vi "Connector 1 DI Engine Sim 2.vi"() -> (3 "Packet":u64)   [LabVIEW 2014]
uses:
  <vilib>/rvi/eio/common/nirviEmuTemplateMethod_errors.vi
  <vilib>/eio/EIONode/EIONode.xnode
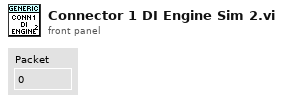
[diagram p1: front panel]
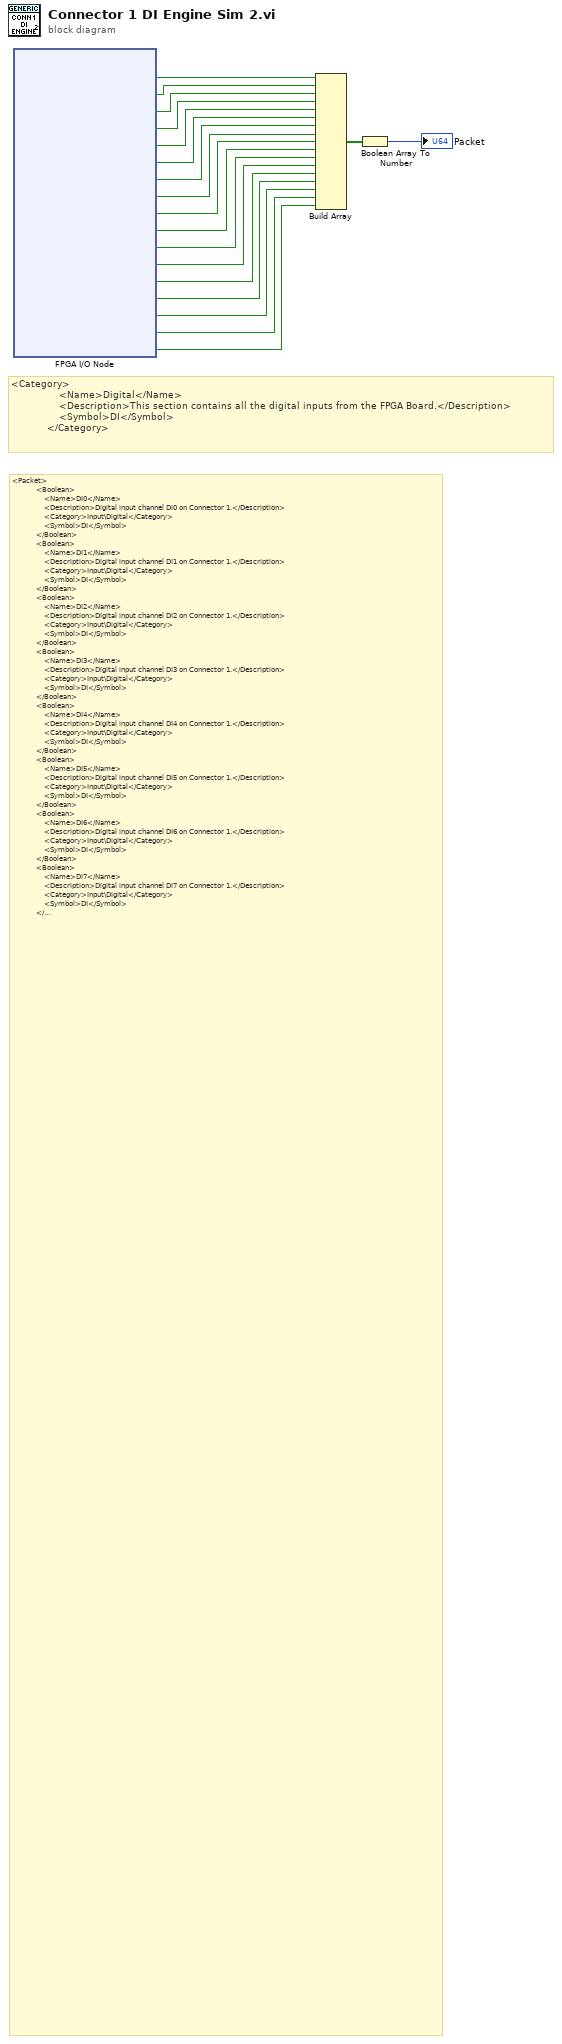
[diagram p0: block diagram]
diagram:
  # "<Packet>\n            <Boolean>\n                <Name>DI0</Name>\n                <Description>Digital input channel DI0 on Connector 1.</Description>\n                <Category>Input\\Digital</Category>\n                <Symbol>DI</Symbol>\n            </Boolean>\n            <Boolean>\n                <Name>DI1</Name>\n                <Description>Digital input channel DI1 on Connector 1.</Description>\n                <Category>Input\\Digital</Category>\n                <Symbol>DI</Symbol>\n            </Boolean>\n            <Boolean>\n                <Name>DI2</Name>\n                <Description>Digital input channel DI2 on Connector 1.</Description>\n                <Category>Input\\Digital</Category>\n                <Symbol>DI</Symbol>\n            </Boolean>\n            <Boolean>\n                <Name>DI3</Name>\n                <Description>Digital input channel DI3 on Connector 1.</Description>\n                <Category>Input\\Digital</Category>\n                <Symbol>DI</Symbol>\n            </Boolean>\n            <Boolean>\n                <Name>DI4</Name>\n                <Description>Digital input channel DI4 on Connector 1.</Description>\n                <Category>Input\\Digital</Category>\n                <Symbol>DI</Symbol>\n            </Boolean>\n            <Boolean>\n                <Name>DI5</Name>\n                <Description>Digital input channel DI5 on Connector 1.</Description>\n                <Category>Input\\Digital</Category>\n                <Symbol>DI</Symbol>\n            </Boolean>\n            <Boolean>\n                <Name>DI6</Name>\n                <Description>Digital input channel DI6 on Connector 1.</Description>\n                <Category>Input\\Digital</Category>\n                <Symbol>DI</Symbol>\n            </Boolean>\n            <Boolean>\n                <Name>DI7</Name>\n                <Description>Digital input channel DI7 on Connector 1.</Description>\n                <Category>Input\\Digital</Category>\n                <Symbol>DI</Symbol>\n            </Boolean>\n            <Boolean>\n                <Name>DI8</Name>\n                <Description>Digital input channel DI8 on Connector 1.</Description>\n                <Category>Input\\Digital</Category>\n                <Symbol>DI</Symbol>\n            </Boolean>\n            <Boolean>\n                <Name>DI9</Name>\n                <Description>Digital input channel DI9 on Connector 1.</Description>\n                <Category>Input\\Digital</Category>\n                <Symbol>DI</Symbol>\n            </Boolean>\n            <Boolean>\n                <Name>DI10</Name>\n                <Description>Digital input channel DI10 on Connector 1.</Description>\n                <Category>Input\\Digital</Category>\n                <Symbol>DI</Symbol>\n            </Boolean>\n            <Boolean>\n                <Name>DI11</Name>\n                <Description>Digital input channel DI11 on Connector 1.</Description>\n                <Category>Input\\Digital</Category>\n                <Symbol>DI</Symbol>\n            </Boolean>\n            <Boolean>\n                <Name>DI12</Name>\n                <Description>Digital input channel DI12 on Connector 1.</Description>\n                <Category>Input\\Digital</Category>\n                <Symbol>DI</Symbol>\n            </Boolean>\n            <Boolean>\n                <Name>DI13</Name>\n                <Description>Digital input channel DI13 on Connector 1.</Description>\n                <Category>Input\\Digital</Category>\n                <Symbol>DI</Symbol>\n            </Boolean>\n            <Boolean>\n                <Name>DI14</Name>\n                <Description>Digital input channel DI14 on Connector 1.</Description>\n                <Category>Input\\Digital</Category>\n                <Symbol>DI</Symbol>\n            </Boolean>\n            <Boolean>\n                <Name>DI15</Name>\n                <Description>Digital input channel DI15 on Connector 1.</Description>\n                <Category>Input\\Digital</Category>\n                <Symbol>DI</Symbol>\n            </Boolean>\n            <Boolean>\n                <Name>DI37</Name>\n                <Description>Digital input channel DI37 on Connector 1.</Description>\n                <Category>Input\\Digital</Category>\n                <Symbol>DI</Symbol>\n            </Boolean>\n        </Packet>"
  # "<Category>\n                <Name>Digital</Name>\n                <Description>This section contains all the digital inputs from the FPGA Board.</Description>\n                <Symbol>DI</Symbol>\n            </Category>"
  n1 = xnode "FPGA I/O Node"() -> ("Connector1/DIO0"=w19:bool, "Connector1/DIO1"=w18:bool, "Connector1/DIO2"=w17:bool, "Connector1/DIO3"=w16:bool, "Connector1/DIO4"=w15:bool, "Connector1/DIO5"=w14:bool, "Connector1/DIO6"=w13:bool, "Connector1/DIO7"=w12:bool, "Connector1/DIO8"=w11:bool, "Connector1/DIO9"=w10:bool, "Connector1/DIO10"=w9:bool, "Connector1/DIO11"=w8:bool, "Connector1/DIO12"=w7:bool, "Connector1/DIO13"=w6:bool, "Connector1/DIO14"=w5:bool, "Connector1/DIO15"=w4:bool, "Connector1/DIO37"=w3:bool)  [unwired: 17 in, 17 out]
  n2 = Build Array(w19, w18, w17, w16, w15, w14, w13, w12, w11, w10, w9, w8, w7, w6, w5, w4, w3) -> (w2:bool[])
  n3 = Boolean Array To Number(Boolean array=w2) -> (number=→"Packet":u32)
